vi "FX29.vi"(11 "Variables and Memory in":T1 {"GFX" format="%02x"}) -> (3 "Variables and Memory out":T1 {"GFX" format="%02x"})   [LabVIEW 2021]
uses:
  Controls/ClusterF.ctl
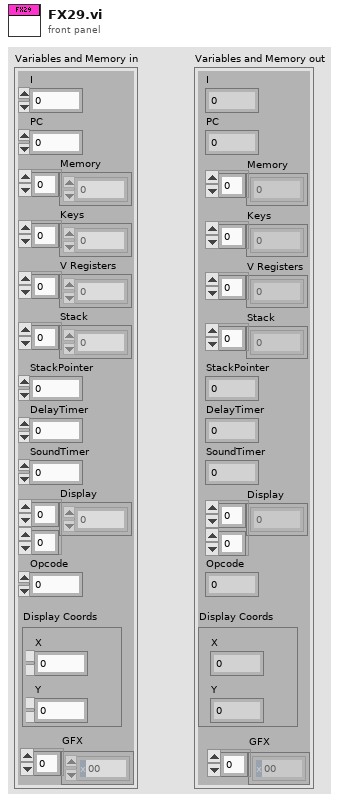
[diagram p1: front panel]
types:
  T1 = typedef "ClusterF.ctl" = cluster{"I":u16, "PC":u16, "Memory":u8[], "Keys":u8[], "V Registers":u8[], "Stack":u16[], "StackPointer":u16, "DelayTimer":u8, "SoundTimer":u8, "Display":u8[][], "Opcode":u16, "Display Coords":cluster{"X":u8, "Y":u8}, "GFX":u8[]}
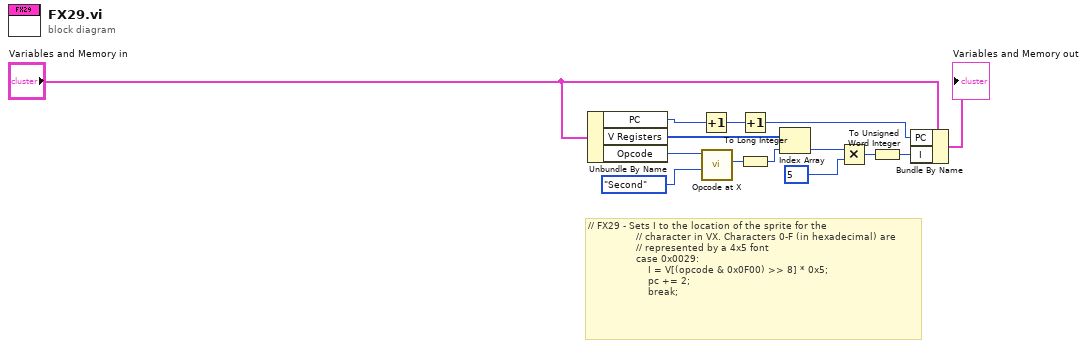
[diagram p0: block diagram]
diagram:
  # "// FX29 - Sets I to the location of the sprite for the\n                // character in VX. Characters 0-F (in hexadecimal) are\n                // represented by a 4x5 font\n                case 0x0029:\n                    I = V[(opcode & 0x0F00) >> 8] * 0x5;\n                    pc += 2;\n                    break;"
  n1 = Unbundle By Name("Variables and Memory in") -> ("PC"=w3:u16, "V Registers"=w8:u8[], "Opcode"=w6:u16)
  n2 = Increment(x=w3) -> (x+1=w4:u16)
  n3 = call "Opcode at X.vi"("X Position"=enum16{"First", "Second", "Third", "Fourth"}."Second", "Opcode"=w6) -> ("Opcode at X Position (U8)"=w9:u8)  [unwired: 9 in]
  n4 = Increment(x=w4) -> (x+1=w5:u16)
  n5 = To Long Integer(number=w9) -> (32bit integer=w10:i32)
  n6 = Index Array(array=w8, index=w10) -> (element=w13:u8)
  n7 = Multiply(x=w13, y=u8 5) -> (x*y=w11:u8)
  n8 = To Unsigned Word Integer(number=w11) -> (unsigned 16bit integer=w12:u16)
  n9 = Bundle By Name(cluster="Variables and Memory in", "PC"=w5, "I"=w12) -> (→"Variables and Memory out":T1)
